vi "RANGE General Data Processing.vi"(0 "DAQ Data Out in":T4, 1 "Meter Select 3":T2, 2 "Meter Select 2":T1, 3 "Meter Select 1":T3, 11 "error in (no error)":errorcluster) -> (4 "DAQ Data Out out":T4, 15 "error out":errorcluster)   [LabVIEW 2016]
uses:
  Type Definitions/RANGE DAQ Data Four Meters.ctl
  Type Definitions/RANGE DAQ Data.ctl
  Drivers/Omega FMA-1600A Series Gas Flow Meter/Type Definitions/FMA1600A Gas Type.ctl
  Drivers/Omega FMA-1600A Series Gas Flow Meter/Type Definitions/FMA1600A Units String.ctl
  Type Definitions/RANGE GAS Data.ctl
  Type Definitions/RANGE Panel Data.ctl
  Type Definitions/RANGE Meter Selector 1-2.ctl
  Type Definitions/RANGE Meter Selector 5-6.ctl
  Type Definitions/RANGE Meter Selector 3-4.ctl
  Type Definitions/Range Meter Bank.ctl
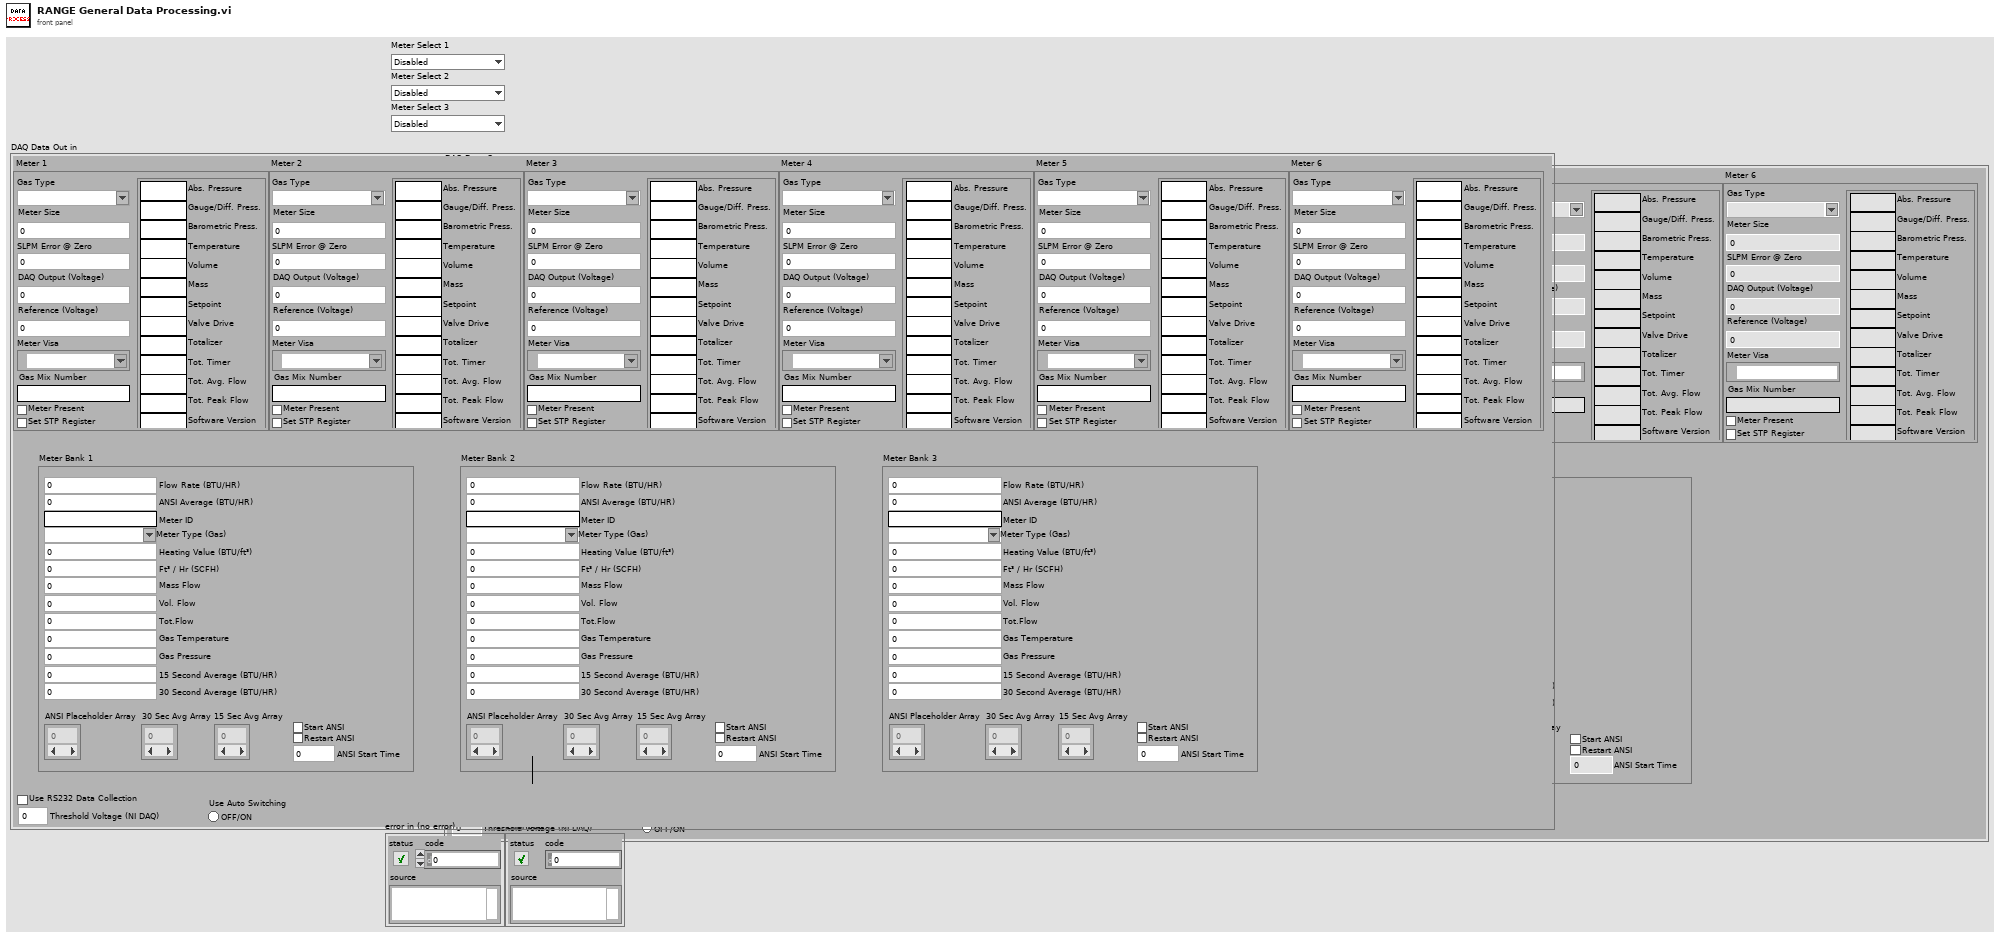
[diagram p1: front panel]
types:
  T1 = typedef "RANGE Meter Selector 3-4.ctl" = enum16{"Disabled", "Meter 3", "Meter 4", "Auto"}
  T2 = typedef "RANGE Meter Selector 5-6.ctl" = enum16{"Disabled", "Meter 5", "Meter 6", "Auto"}
  T3 = typedef "RANGE Meter Selector 1-2.ctl" = enum16{"Disabled", "Meter 1", "Meter 2", "Auto"}
  T4 = typedef "RANGE DAQ Data Four Meters.ctl" = cluster{"Meter 1":T5, "Meter 2":T5, "Meter 3":T5, "Meter 4":T5, "Meter 5":T5, "Meter 6":T5, "Meter Bank 1":T8, "Meter Bank 2":T8, "Meter Bank 3":T8, "Threshold Voltage (NI DAQ)":dbl, "Use RS232 Data Collection":bool, "Use Auto Switching":bool}
  T5 = typedef "RANGE DAQ Data.ctl" = cluster{"Meter Size":dbl, "DAQ Output (Voltage)":dbl, "Reference (Voltage)":dbl, "Meter Present":bool, "Meter Visa":refnum<visa-resource-name>, "Gas Type":T6, "SLPM Error @ Zero":dbl, "Gas Mix Number":string, "Set STP Register":bool, "Measurement Units":T7}
  T6 = typedef "FMA1600A Gas Type.ctl" = string
  T7 = typedef "FMA1600A Units String.ctl" = cluster{"Abs. Pressure":string, "Gauge/Diff. Press.":string, "Barometric Press.":string, "Temperature":string, "Volume":string, "Mass":string, "Setpoint":string, "Valve Drive":string, "Totalizer":string, "Tot. Timer":string, "Tot. Avg. Flow":string, "Tot. Peak Flow":string, "Software Version":string}
  T8 = typedef "RANGE GAS Data.ctl" = cluster{"Flow Rate (BTU/HR)":dbl, "ANSI Placeholder Array":dbl[], "15 Sec Avg Array":dbl[], "30 Sec Avg Array ":dbl[], "ANSI Average (BTU/HR)":dbl, "Panel Data":T9, "Start ANSI":bool, "ANSI Start Time":dbl, "Restart ANSI":bool, "Meter ID":string}
  T9 = typedef "RANGE Panel Data.ctl" = cluster{"Meter Type (Gas)":T6, "Heating Value (BTU/ft³)":dbl, "Ft³ / Hr (SCFH)":dbl, "15 Second Average (BTU/HR)":dbl, "30 Second Average (BTU/HR)":dbl, "Mass Flow":dbl, "Vol. Flow":dbl, "Gas Temperature":dbl, "Gas Pressure":dbl, "Tot.Flow":dbl}
  T10 = typedef "Range Meter Bank.ctl" = enum16{"Meter Bank 1", "Meter Bank 2", "Meter Bank 3"}
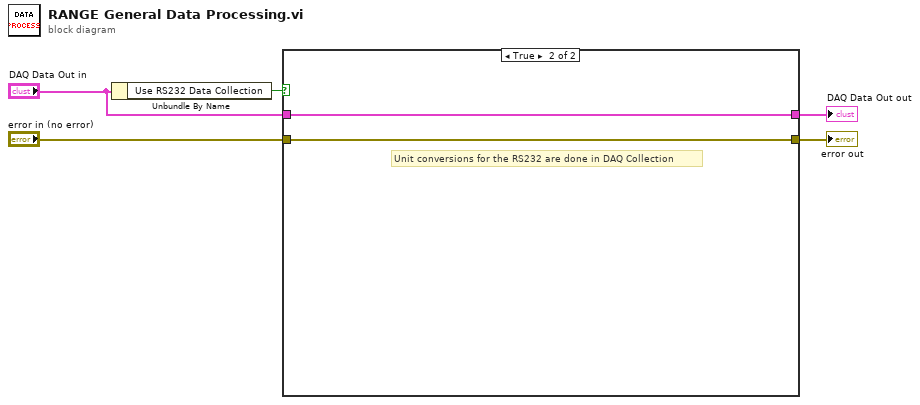
[diagram p0: block diagram]
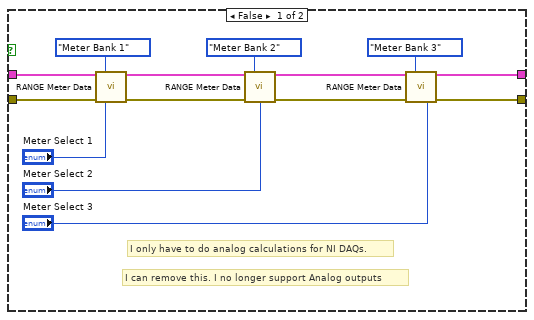
[diagram p2: hidden frame]
diagram:
  n1 = Unbundle By Name("DAQ Data Out in") -> ("Use RS232 Data Collection"=w3:bool)
  n2 = case shown="True" w3 {
    tunnel: [w19 w21] -> w2
    tunnel: [w16 w20] -> w1
    tunnel: "DAQ Data Out in" -> [w14 w21]
    tunnel: "error in (no error)" -> [w12 w20]
    frame False {
      # "I can remove this. I no longer support Analog outputs"
      # "I only have to do analog calculations for NI DAQs."
      n3 = call "RANGE Meter Data.vi"("DAQ Data"=w14, "Meter Number"=Range_Meter_Bank."Meter Bank 1", "Error In"=w12, "Meter Select 1"="Meter Select 1") -> ("DAQ Data Out"=w17:T4, "Error Out"=w13:errorcluster)  [unwired: 10 in]
      n4 = call "RANGE Meter Data.vi"("DAQ Data"=w17, "Meter Number"=Range_Meter_Bank."Meter Bank 2", "Error In"=w13, "Meter Select 2"="Meter Select 2") -> ("DAQ Data Out"=w18:T4, "Error Out"=w15:errorcluster)  [unwired: 10 in]
      n5 = call "RANGE Meter Data.vi"("DAQ Data"=w18, "Meter Number"=Range_Meter_Bank."Meter Bank 3", "Error In"=w15, "Meter Select 3"="Meter Select 3") -> ("DAQ Data Out"=w19:T4, "Error Out"=w16:errorcluster)  [unwired: 10 in]
    }
    frame True {
      # "Unit conversions for the RS232 are done in DAQ Collection"
    }
  }
  "DAQ Data Out out" <- w2
  "error out" <- w1
